vi "Save File Dialog with Overwrite Option.vi"(6 "prompt":string, 7 "Default Name":string, 8 "error in (no error)":errorcluster, 9 "pattern label":string, 10 "pattern (all files)":string, 11 "Starting Folder":path) -> (0 "error out":errorcluster, 1 "overwritten":bool, 2 "cancelled":bool, 3 "selected path":path)   [LabVIEW 2021, in "Files.lvlib"]
uses:
  Files.lvlib
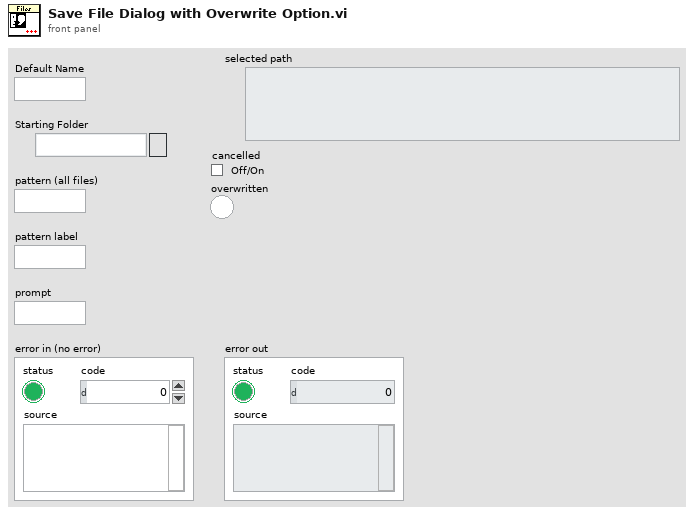
[diagram p1: front panel]
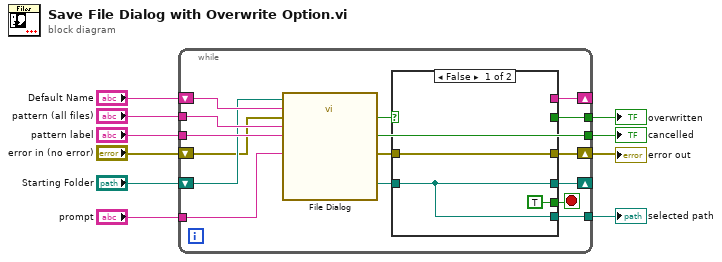
[diagram p0: block diagram]
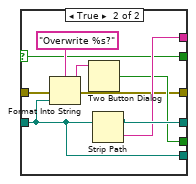
[diagram p2: hidden frame]
diagram:
  n1 = while {
    tunnel: "pattern label" -> [w25]
    tunnel: "pattern (all files)" -> [w24]
    tunnel: [w23] -> w7
    tunnel: "prompt" -> [w20]
    shift-right: [w15] -> _
    shift-left: "Starting Folder" -> [w22]
    shift-right: [w17] -> w4
    shift-left: "error in (no error)" -> [w21]
    shift-right: [w14] -> _
    shift-left: "Default Name" -> [w26]
    tunnel: [w13] -> w2
    tunnel: [w11] -> w1
    stop <- w12 stop-if-true
    n2 = call "File Dialog"("start path"=w22, "prompt"=w20, "default name"=w26, "error in"=w21, "pattern (all files)"=w24, "pattern label"=w25) -> ("selected path"=w16:path, "exists"=w19:bool, "cancelled"=w23:bool, "error out"=w18:errorcluster)  [unwired: 6 in]
    n3 = case shown="False" w19 {
      selector: w19 -> [_ w30]
      tunnel: w18 -> [w29 w34]
      tunnel: [w29 w31] -> w17
      tunnel: w16 -> [w28 w33]
      tunnel: [w28 w38] -> w15
      tunnel: [_ w37] -> w14
      tunnel: [w28 w33] -> w13
      tunnel: [TRUE w32] -> w12
      tunnel: [_ w30] -> w11
      frame False {
      }
      frame True {
        n4 = Format Into String(format string="Overwrite %s?", error in=w34, w33) -> (resulting string=w36:string, error out=w31:errorcluster)  [unwired: 1 in]
        n5 = Two Button Dialog(message=w36) -> (T button?=w32:bool)  [unwired: 2 in]
        n6 = Strip Path(path=w33) -> (stripped path=w38:path, name=w37:string)
      }
    }
  }
  "cancelled" <- w7
  "error out" <- w4
  "selected path" <- w2
  "overwritten" <- w1
